vi "IMAQ sum.vi"(11 "Image":T1) -> (3 "Sum":i32)   [LabVIEW 2012, in "LightPipes.lvlib"]
uses:
  LightPipes.lvlib
  <vilib>/vision/Image Controls.llb/IMAQ Image.ctl
panel:
  # "Sum up pixel intensity of an image"
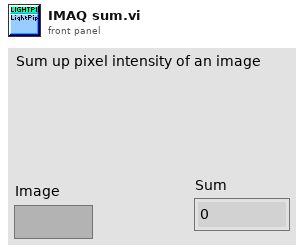
[diagram p1: front panel]
types:
  T1 = typedef "IMAQ Image.ctl" = refnum<image>
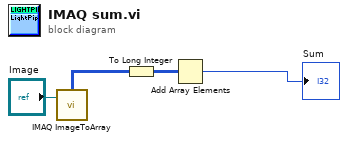
[diagram p0: block diagram]
diagram:
  n1 = call "IMAQ ImageToArray"("Image"="Image") -> ("Image Pixels (U8)"=w3:u8[][])  [unwired: 3 in, 4 out]
  n2 = To Long Integer(number=w3) -> (32bit integer=w1:i32[][])
  n3 = Add Array Elements(numeric array=w1) -> (sum=→"Sum":i32)
